vi "Red targets.vi"(11 "cluster":cluster{dbl, dbl, dbl}) -> (3 "Array":T1[](array[typedef]))   [LabVIEW 2010]
uses:
  <vilib>/Utility/miscctls.llb/LVRGBAColorTypeDef.ctl
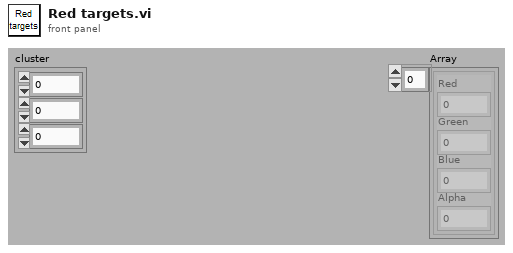
[diagram p1: front panel]
types:
  T1 = typedef "LVRGBAColorTypeDef.ctl" = cluster{"Red":sgl, "Green":sgl, "Blue":sgl, "Alpha":sgl}
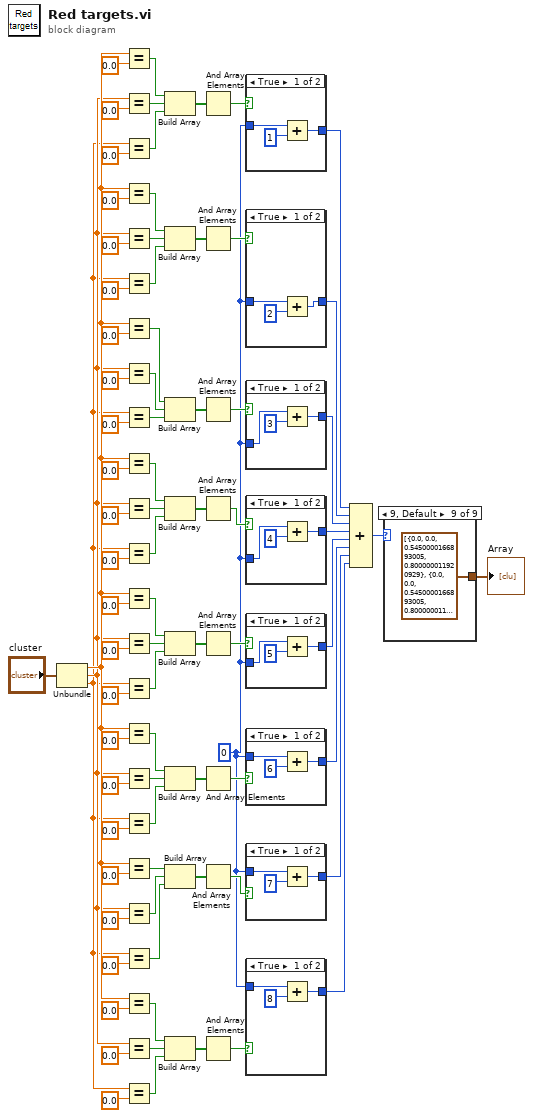
[diagram p0: block diagram]
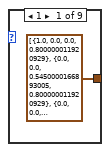
[diagram p2: hidden frame]
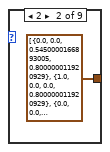
[diagram p3: hidden frame]
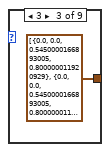
[diagram p4: hidden frame]
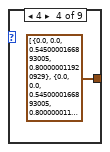
[diagram p5: hidden frame]
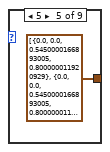
[diagram p6: hidden frame]
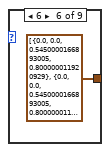
[diagram p7: hidden frame]
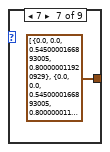
[diagram p8: hidden frame]
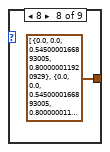
[diagram p9: hidden frame]
diagram:
  w11 = 0 ("Scrolling")
  n1 = Unbundle("cluster") -> (w78:dbl, w77:dbl, w76:dbl)
  n2 = Equal?(x=w78, y=0.0) -> (x = y?=w51:bool)
  n3 = Equal?(x=w77, y=0.0) -> (x = y?=w50:bool)
  n4 = Equal?(x=w76, y=0.0) -> (x = y?=w49:bool)
  n5 = Equal?(x=w78, y=0.0) -> (x = y?=w46:bool)
  n6 = Equal?(x=w77, y=0.0) -> (x = y?=w45:bool)
  n7 = Equal?(x=w76, y=0.0) -> (x = y?=w44:bool)
  n8 = Equal?(x=w78, y=0.0) -> (x = y?=w42:bool)
  n9 = Equal?(x=w77, y=0.0) -> (x = y?=w41:bool)
  n10 = Equal?(x=w76, y=0.0) -> (x = y?=w40:bool)
  n11 = Equal?(x=w78, y=0.0) -> (x = y?=w37:bool)
  n12 = Equal?(x=w77, y=0.0) -> (x = y?=w36:bool)
  n13 = Equal?(x=w76, y=0.0) -> (x = y?=w35:bool)
  n14 = Equal?(x=w78, y=0.0) -> (x = y?=w32:bool)
  n15 = Equal?(x=w77, y=0.0) -> (x = y?=w31:bool)
  n16 = Equal?(x=w76, y=0.0) -> (x = y?=w30:bool)
  n17 = Equal?(x=w78, y=0.0) -> (x = y?=w27:bool)
  n18 = Equal?(x=w77, y=0.0) -> (x = y?=w26:bool)
  n19 = Equal?(x=w76, y=0.0) -> (x = y?=w25:bool)
  n20 = Equal?(x=w78, y=0.0) -> (x = y?=w22:bool)
  n21 = Equal?(x=w77, y=0.0) -> (x = y?=w21:bool)
  n22 = Equal?(x=w76, y=0.0) -> (x = y?=w20:bool)
  n23 = Equal?(x=w78, y=0.0) -> (x = y?=w17:bool)
  n24 = Equal?(x=w77, y=0.0) -> (x = y?=w16:bool)
  n25 = Equal?(x=w76, y=0.0) -> (x = y?=w15:bool)
  n26 = Build Array(w51, w50, w49) -> (w48:bool[])
  n27 = Build Array(w46, w45, w44) -> (w43:bool[])
  n28 = Build Array(w42, w41, w40) -> (w39:bool[])
  n29 = Build Array(w37, w36, w35) -> (w34:bool[])
  n30 = Build Array(w32, w31, w30) -> (w29:bool[])
  n31 = Build Array(w27, w26, w25) -> (w24:bool[])
  n32 = Build Array(w22, w21, w20) -> (w19:bool[])
  n33 = Build Array(w17, w16, w15) -> (w14:bool[])
  n34 = And Array Elements(Boolean array=w48) -> (logical AND=w47:bool)
  n35 = And Array Elements(Boolean array=w43) -> (logical AND=w12:bool)
  n36 = And Array Elements(Boolean array=w39) -> (logical AND=w38:bool)
  n37 = And Array Elements(Boolean array=w34) -> (logical AND=w33:bool)
  n38 = And Array Elements(Boolean array=w29) -> (logical AND=w28:bool)
  n39 = And Array Elements(Boolean array=w24) -> (logical AND=w23:bool)
  n40 = And Array Elements(Boolean array=w19) -> (logical AND=w18:bool)
  n41 = And Array Elements(Boolean array=w14) -> (logical AND=w13:bool)
  n42 = case shown="True" w47 {
    tunnel: w11 -> [w82 w83]
    tunnel: [w80 w83] -> w10
    frame True {
      n43 = Add(x=w82, y=1) -> (x+y=w80:i32)
    }
    frame False {
    }
  }
  n44 = case shown="True" w12 {
    tunnel: w11 -> [w85 w87]
    tunnel: [w84 w87] -> w9
    frame True {
      n45 = Add(x=w85, y=2) -> (x+y=w84:i32)
    }
    frame False {
    }
  }
  n46 = case shown="True" w38 {
    tunnel: w11 -> [w89 w91]
    tunnel: [w88 w91] -> w8
    frame True {
      n47 = Add(x=w89, y=3) -> (x+y=w88:i32)
    }
    frame False {
    }
  }
  n48 = case shown="True" w33 {
    tunnel: w11 -> [w93 w95]
    tunnel: [w92 w95] -> w7
    frame True {
      n49 = Add(x=w93, y=4) -> (x+y=w92:i32)
    }
    frame False {
    }
  }
  n50 = case shown="True" w28 {
    tunnel: w11 -> [w97 w99]
    tunnel: [w96 w99] -> w6
    frame True {
      n51 = Add(x=w97, y=5) -> (x+y=w96:i32)
    }
    frame False {
    }
  }
  n52 = case shown="True" w23 {
    tunnel: w11 -> [w101 w103]
    tunnel: [w100 w103] -> w5
    frame True {
      n53 = Add(x=w101, y=6) -> (x+y=w100:i32)
    }
    frame False {
    }
  }
  n54 = case shown="True" w18 {
    tunnel: w11 -> [w105 w107]
    tunnel: [w104 w107] -> w4
    frame True {
      n55 = Add(x=w105, y=7) -> (x+y=w104:i32)
    }
    frame False {
    }
  }
  n56 = case shown="True" w13 {
    tunnel: w11 -> [w109 w111]
    tunnel: [w108 w111] -> w3
    frame True {
      n57 = Add(x=w109, y=8) -> (x+y=w108:i32)
    }
    frame False {
    }
  }
  n58 = Compound Arithmetic op=ADD(w10, w9, w8, w7, w6, w5, w4, w3) -> (w2:i32)
  n59 = case shown="9, Default" w2 {
    tunnel: [T1[] [{"Red"=1.0, "Green"=0.0, "Blue"=0.0, "Alpha"=0.8}, {"Red"=0.0, "Green"=0.0, "Blue"=0.545, "Alpha"=0.8}, {"Red"=0.0, "Green"=0.0, "Blue"=0.545, "Alpha"=0.8}, {"Red"=0.0, "Green"=0.0, "Blue"=0.545, "Alpha"=0.8}, {"Red"=0.0, "Green"=0.0, "Blue"=0.545, "Alpha"=0.8}, {"Red"=0.0, "Green"=0.0, "Blue"=0.545, "Alpha"=0.8}, {"Red"=0.0, "Green"=0.0, "Blue"=0.545, "Alpha"=0.8}, {"Red"=0.0, "Green"=0.0, "Blue"=0.545, "Alpha"=0.8}] ("Array") T1[] [{"Red"=0.0, "Green"=0.0, "Blue"=0.545, "Alpha"=0.8}, {"Red"=1.0, "Green"=0.0, "Blue"=0.0, "Alpha"=0.8}, {"Red"=0.0, "Green"=0.0, "Blue"=0.545, "Alpha"=0.8}, {"Red"=0.0, "Green"=0.0, "Blue"=0.545, "Alpha"=0.8}, {"Red"=0.0, "Green"=0.0, "Blue"=0.545, "Alpha"=0.8}, {"Red"=0.0, "Green"=0.0, "Blue"=0.545, "Alpha"=0.8}, {"Red"=0.0, "Green"=0.0, "Blue"=0.545, "Alpha"=0.8}, {"Red"=0.0, "Green"=0.0, "Blue"=0.545, "Alpha"=0.8}] ("Array") T1[] [{"Red"=0.0, "Green"=0.0, "Blue"=0.545, "Alpha"=0.8}, {"Red"=0.0, "Green"=0.0, "Blue"=0.545, "Alpha"=0.8}, {"Red"=1.0, "Green"=0.0, "Blue"=0.0, "Alpha"=0.8}, {"Red"=0.0, "Green"=0.0, "Blue"=0.545, "Alpha"=0.8}, {"Red"=0.0, "Green"=0.0, "Blue"=0.545, "Alpha"=0.8}, {"Red"=0.0, "Green"=0.0, "Blue"=0.545, "Alpha"=0.8}, {"Red"=0.0, "Green"=0.0, "Blue"=0.545, "Alpha"=0.8}, {"Red"=0.0, "Green"=0.0, "Blue"=0.545, "Alpha"=0.8}] ("Array") T1[] [{"Red"=0.0, "Green"=0.0, "Blue"=0.545, "Alpha"=0.8}, {"Red"=0.0, "Green"=0.0, "Blue"=0.545, "Alpha"=0.8}, {"Red"=0.0, "Green"=0.0, "Blue"=0.545, "Alpha"=0.8}, {"Red"=1.0, "Green"=0.0, "Blue"=0.0, "Alpha"=0.8}, {"Red"=0.0, "Green"=0.0, "Blue"=0.545, "Alpha"=0.8}, {"Red"=0.0, "Green"=0.0, "Blue"=0.545, "Alpha"=0.8}, {"Red"=0.0, "Green"=0.0, "Blue"=0.545, "Alpha"=0.8}, {"Red"=0.0, "Green"=0.0, "Blue"=0.545, "Alpha"=0.8}] ("Array") T1[] [{"Red"=0.0, "Green"=0.0, "Blue"=0.545, "Alpha"=0.8}, {"Red"=0.0, "Green"=0.0, "Blue"=0.545, "Alpha"=0.8}, {"Red"=0.0, "Green"=0.0, "Blue"=0.545, "Alpha"=0.8}, {"Red"=0.0, "Green"=0.0, "Blue"=0.545, "Alpha"=0.8}, {"Red"=1.0, "Green"=0.0, "Blue"=0.0, "Alpha"=0.8}, {"Red"=0.0, "Green"=0.0, "Blue"=0.545, "Alpha"=0.8}, {"Red"=0.0, "Green"=0.0, "Blue"=0.545, "Alpha"=0.8}, {"Red"=0.0, "Green"=0.0, "Blue"=0.545, "Alpha"=0.8}] ("Array") T1[] [{"Red"=0.0, "Green"=0.0, "Blue"=0.545, "Alpha"=0.8}, {"Red"=0.0, "Green"=0.0, "Blue"=0.545, "Alpha"=0.8}, {"Red"=0.0, "Green"=0.0, "Blue"=0.545, "Alpha"=0.8}, {"Red"=0.0, "Green"=0.0, "Blue"=0.545, "Alpha"=0.8}, {"Red"=0.0, "Green"=0.0, "Blue"=0.545, "Alpha"=0.8}, {"Red"=1.0, "Green"=0.0, "Blue"=0.0, "Alpha"=0.8}, {"Red"=0.0, "Green"=0.0, "Blue"=0.545, "Alpha"=0.8}, {"Red"=0.0, "Green"=0.0, "Blue"=0.545, "Alpha"=0.8}] ("Array") T1[] [{"Red"=0.0, "Green"=0.0, "Blue"=0.545, "Alpha"=0.8}, {"Red"=0.0, "Green"=0.0, "Blue"=0.545, "Alpha"=0.8}, {"Red"=0.0, "Green"=0.0, "Blue"=0.545, "Alpha"=0.8}, {"Red"=0.0, "Green"=0.0, "Blue"=0.545, "Alpha"=0.8}, {"Red"=0.0, "Green"=0.0, "Blue"=0.545, "Alpha"=0.8}, {"Red"=0.0, "Green"=0.0, "Blue"=0.545, "Alpha"=0.8}, {"Red"=1.0, "Green"=0.0, "Blue"=0.0, "Alpha"=0.8}, {"Red"=0.0, "Green"=0.0, "Blue"=0.545, "Alpha"=0.8}] ("Array") T1[] [{"Red"=0.0, "Green"=0.0, "Blue"=0.545, "Alpha"=0.8}, {"Red"=0.0, "Green"=0.0, "Blue"=0.545, "Alpha"=0.8}, {"Red"=0.0, "Green"=0.0, "Blue"=0.545, "Alpha"=0.8}, {"Red"=0.0, "Green"=0.0, "Blue"=0.545, "Alpha"=0.8}, {"Red"=0.0, "Green"=0.0, "Blue"=0.545, "Alpha"=0.8}, {"Red"=0.0, "Green"=0.0, "Blue"=0.545, "Alpha"=0.8}, {"Red"=0.0, "Green"=0.0, "Blue"=0.545, "Alpha"=0.8}, {"Red"=1.0, "Green"=0.0, "Blue"=0.0, "Alpha"=0.8}] ("Array") T1[] [{"Red"=0.0, "Green"=0.0, "Blue"=0.545, "Alpha"=0.8}, {"Red"=0.0, "Green"=0.0, "Blue"=0.545, "Alpha"=0.8}, {"Red"=0.0, "Green"=0.0, "Blue"=0.545, "Alpha"=0.8}, {"Red"=0.0, "Green"=0.0, "Blue"=0.545, "Alpha"=0.8}, {"Red"=0.0, "Green"=0.0, "Blue"=0.545, "Alpha"=0.8}, {"Red"=0.0, "Green"=0.0, "Blue"=0.545, "Alpha"=0.8}, {"Red"=0.0, "Green"=0.0, "Blue"=0.545, "Alpha"=0.8}, {"Red"=0.0, "Green"=0.0, "Blue"=0.545, "Alpha"=0.8}] ("Array")] -> w1
    frame 1 {
    }
    frame 2 {
    }
    frame 3 {
    }
    frame 4 {
    }
    frame 5 {
    }
    frame 6 {
    }
    frame 7 {
    }
    frame 8 {
    }
    frame 9, Default {
    }
  }
  "Array" <- w1
